vi "meth.SetStreamReader.vi"(0 "class.GLue in":refnum<class "class.GLue.lvclass">, 2 "StreamReader":refnum<vi>, 5 "UserData":variant, 11 "error in":errorcluster, 13 "ms timeout (-1)":i32=-1) -> (4 "class.GLue out":refnum<class "class.GLue.lvclass">, 15 "error out":errorcluster)   [LabVIEW 2014, in "GLue.lvlib" / "class.GLue.lvclass"]
uses:
  class.GLue.lvclass
  class.GLue.lvclass/class.GLue.ctl
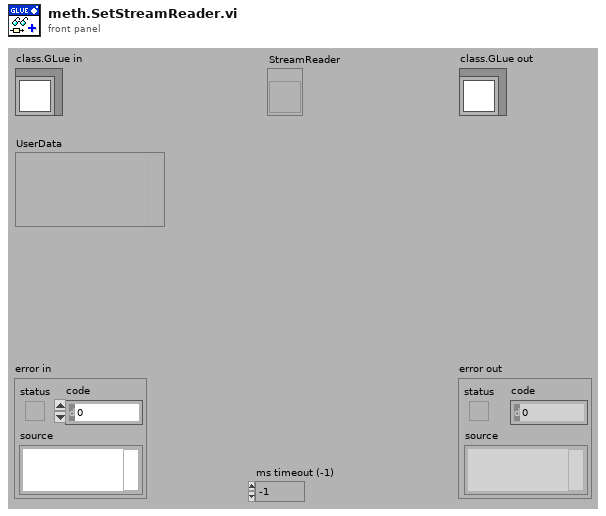
[diagram p1: front panel]
types:
  T1 = typedef "Semaphore RefNum" = refnum<k1>
  T2 = cluster{"StreamReader":refnum<vi>, "UserData":variant}
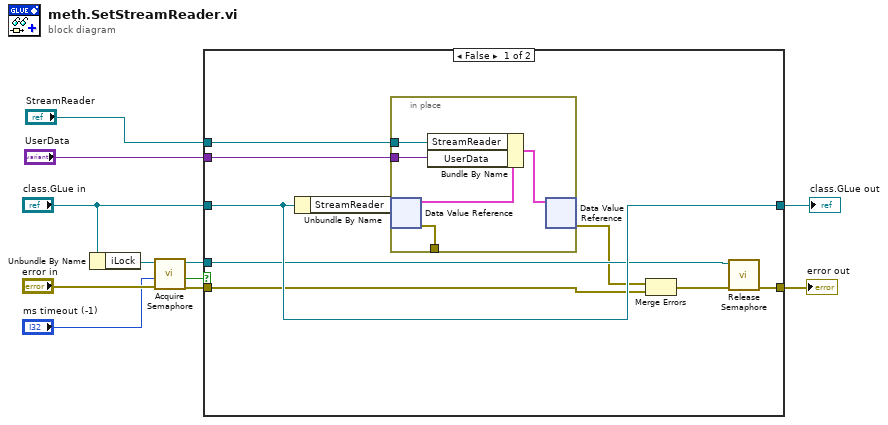
[diagram p0: block diagram]
diagram:
  n1 = Unbundle By Name("class.GLue in") -> ("iLock"=w11:T1)
  n2 = call <vilib>:"Acquire Semaphore.vi"("error in (no error)"="error in", "ms timeout (-1)"="ms timeout (-1)", "semaphore"=w11) -> ("error out"=w10:errorcluster, "timed out"=w9:bool, "semaphore out"=w8:T1)  [unwired: 2 in]
  n3 = case shown="False" w9 {
    tunnel: [w20 w26] -> w3
    tunnel: [w19 w27] -> w4
    tunnel: "class.GLue in" -> [w19 w27]
    tunnel: w10 -> [w18 w26]
    tunnel: w8 -> [w16 _]
    tunnel: "StreamReader" -> [w13 _]
    tunnel: "UserData" -> [w12 _]
    frame False {
      n4 = Unbundle By Name(w19) -> ("StreamReader"=w15:refnum<data-value>)
      n5 = in-place {
        in-place-border: [w25] -> _
        in-place-border: w13 -> [w22]
        in-place-border: w12 -> [w21]
        n6 = in-place-dvr #1(w15) -> (w24:T2, w25:errorcluster)
        n7 = Bundle By Name(cluster=w24, "StreamReader"=w22, "UserData"=w21) -> (w23:T2)
        n8 = in-place-dvr #1(w23) -> (w14:errorcluster)  [unwired: 1 out]
      }
      n9 = Merge Errors(w14, w18) -> (w17:errorcluster)
      n10 = call <vilib>:"Release Semaphore.vi"("error in (no error)"=w17, "semaphore"=w16) -> ("error out"=w20:errorcluster)  [unwired: 4 in, 1 out]
    }
    frame True {
    }
  }
  "error out" <- w3
  "class.GLue out" <- w4
